vi "replaceYearMonthToken.vi"(8 "error in (no error)":errorcluster, 10 "Querry In":string, 11 "Goal in":refnum<class "Goal.lvclass">) -> (0 "error out":errorcluster, 2 "Query Out":string, 3 "Goal out":refnum<class "Goal.lvclass">)   [LabVIEW 2018, in "Goal.lvclass"]
uses:
  Goal.lvclass
  Goal.lvclass/Goal.ctl
  WhichMonth/WhichMonth.lvclass
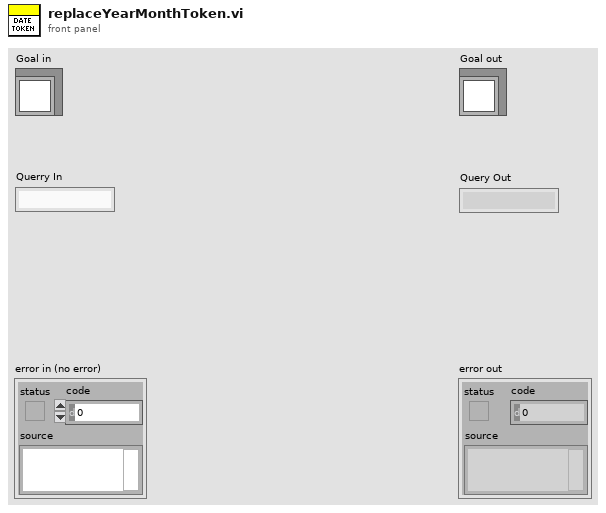
[diagram p1: front panel]
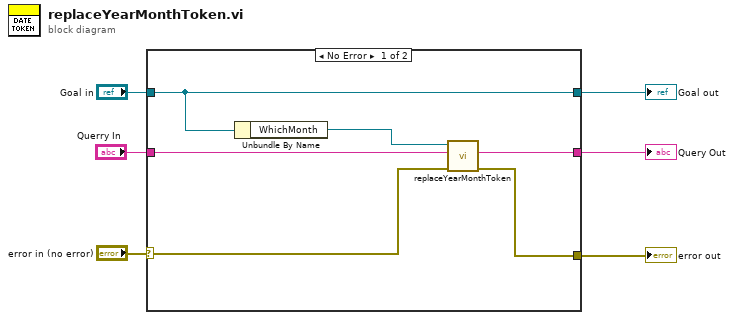
[diagram p0: block diagram]
diagram:
  n1 = case shown="No Error" "error in (no error)" {
    selector: "error in (no error)" -> [w8 w14]
    tunnel: [w9 w14] -> w5
    tunnel: [w12 w13] -> w3
    tunnel: "Goal in" -> [w12 w13]
    tunnel: [w10 _] -> w2
    tunnel: "Querry In" -> [w11 _]
    frame No Error {
      n2 = Unbundle By Name(w12) -> ("WhichMonth"=w7:refnum<class "WhichMonth.lvclass">)
      n3 = call "replaceYearMonthToken.vi"("error in (no error)"=w8, "Query In"=w11, "WhichMonth in"=w7) -> ("error out"=w9:errorcluster, "Query Out"=w10:string)  [unwired: 6 in, 1 out]
    }
    frame Error {
    }
  }
  "error out" <- w5
  "Goal out" <- w3
  "Query Out" <- w2
